vi "Read Command.vi"(8 "error in (no error)":errorcluster, 10 "Command Data":T1, 11 "F4T in":refnum<class "F4T.lvclass">) -> (0 "error out":errorcluster, 2 "Response":string, 3 "F4T out":refnum<class "F4T.lvclass">)   [LabVIEW 2018, in "F4T.lvlib" / "F4T.lvclass"]
doc: "Read Command for Watlow F4T."
uses:
  F4T.lvclass
  Custom Controls/Command Data.ctl
  F4T.lvclass/F4T.ctl
  C:/Program Files/National Instruments/LabVIEW 2018/instr.lib/Watlow Std Bus/Public/Watbus.dll
  Program Files/National Instruments/LabVIEW 2018/instr.lib/Watlow Std Bus/Public/Watbus.dll
  PPLs/Temp Chamber/Parent/Temp Chamber.lvlibp/Temp Chamber.lvclass
  C:/Projects/LabVIEW/PPLs/Temp Chamber/Parent/Temp Chamber.lvlibp/Temp Chamber.lvclass
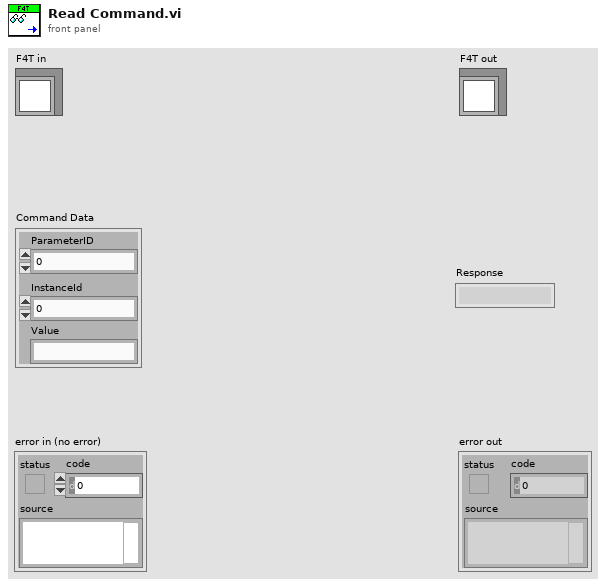
[diagram p1: front panel]
types:
  T1 = typedef "F4T.lvlib/F4T.lvclass/Command Data.ctl" = cluster{"ParameterID":u32, "InstanceId":u32, "Value":string}
  T2 = typedef "Temp Chamber.lvlibp/Temp Chamber.lvclass/Temp Units.ctl" = enum16{"Celsius", "Fahrenheit", "Kelvin", "Rankine"}
  T3 = typedef "F4T.lvlib/F4T.lvclass/Control Data.ctl" = cluster{"DeviceType ":u32, "Zone":u32}
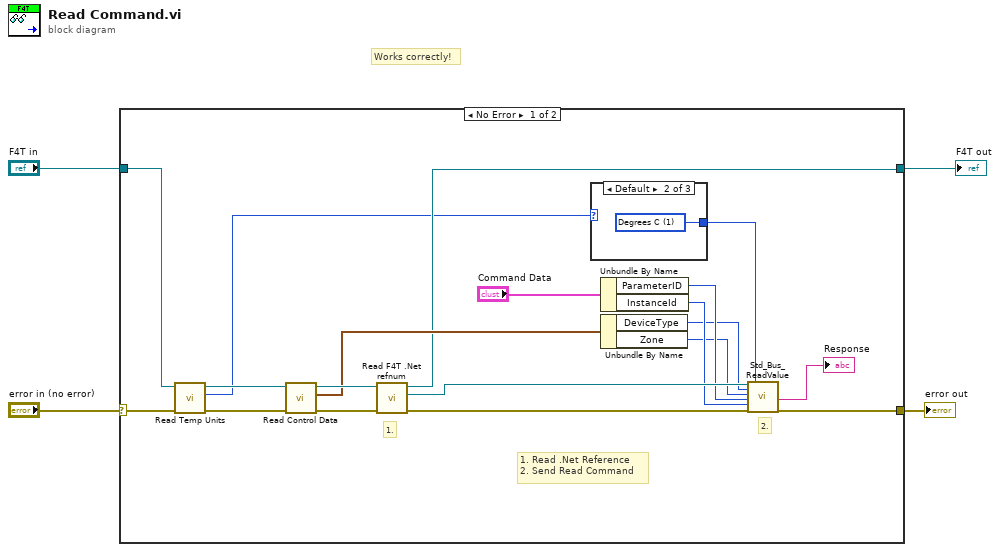
[diagram p0: block diagram]
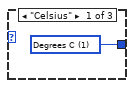
[diagram p2: hidden frame]
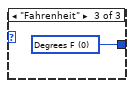
[diagram p3: hidden frame]
diagram:
  # "Works correctly!"
  n1 = case shown="No Error" "error in (no error)" {
    selector: "error in (no error)" -> [w8 w28]
    tunnel: [w12 w28] -> w3
    tunnel: [w11 w27] -> w1
    tunnel: "F4T in" -> [w9 w27]
    frame No Error {
      # "1. Read .Net Reference\n2. Send Read Command"
      # "2."
      # "1."
      n2 = call "Read Temp Units.vi"("error in (no error)"=w8, "Temp Chamber in"=w9) -> ("error out"=w6:errorcluster, "Temp Units"=w5:T2, "Temp Chamber out"=w7:refnum<class "F4T.lvclass">)  [unwired: 7 in]
      n3 = call "Read Control Data.vi"("error in (no error)"=w6, "F4T in"=w7) -> ("error out"=w17:errorcluster, "Control Data"=w15:T3, "F4T out"=w16:refnum<class "F4T.lvclass">)  [unwired: 7 in]
      n4 = call "Read F4T .Net refnum.vi"("error in (no error)"=w17, "F4T in"=w16) -> ("error out"=w23:errorcluster, "F4T .Net refnum"=w21:refnum<k24>, "F4T out"=w11:refnum<class "F4T.lvclass">)  [unwired: 7 in]
      n5 = case shown="Default" w5 {
        tunnel: [w24 w25 w26] -> w10
        frame "Celsius" {
          w24 = u8 1 items=["Degrees F", "Degrees C"] ("TemperatureUnits")
        }
        frame Default {
          w25 = u8 1 items=["Degrees F", "Degrees C"] ("TemperatureUnits")
        }
        frame "Fahrenheit" {
          w26 = u8 0 items=["Degrees F", "Degrees C"] ("TemperatureUnits")
        }
      }
      n6 = Unbundle By Name("Command Data") -> ("ParameterID"=w19:u32, "InstanceId"=w18:u32)
      n7 = Unbundle By Name(w15) -> ("DeviceType"=w14:u32, "Zone"=w13:u32)
      n8 = call <instrlib>:"Std_Bus_ReadValue.vi"("ILabVIEW In"=w21, "DeviceType"=w14, "Zone"=w13, "ParameterID"=w19, "InstanceId"=w18, "error in (no error)"=w23, "TemperatureUnits"=w10) -> ("Value Out"=→"Response":string, "error out"=w12:errorcluster)  [unwired: 10 in, 1 out]
    }
    frame Error {
    }
  }
  "error out" <- w3
  "F4T out" <- w1
